vi "xy_graph_copy_format-vertical.vi"(6 "xy_scales_to_copy":i32=1, 8 "error in (no error)":errorcluster, 10 "destination":refnum<vi>, 11 "source":refnum<vi>) -> (0 "error out":errorcluster)   [LabVIEW 2015, in "lv-graph.lvlib"]
uses:
  lv-graph.lvlib
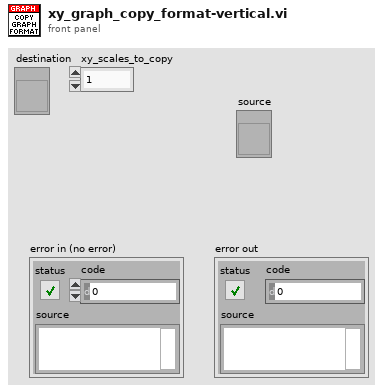
[diagram p1: front panel]
types:
  T1 = typedef "LVRangeTypeDef.ctl" = cluster{"Minimum":dbl, "Maximum":dbl, "Increment":dbl, "Minor Increment":dbl, "Start":dbl}
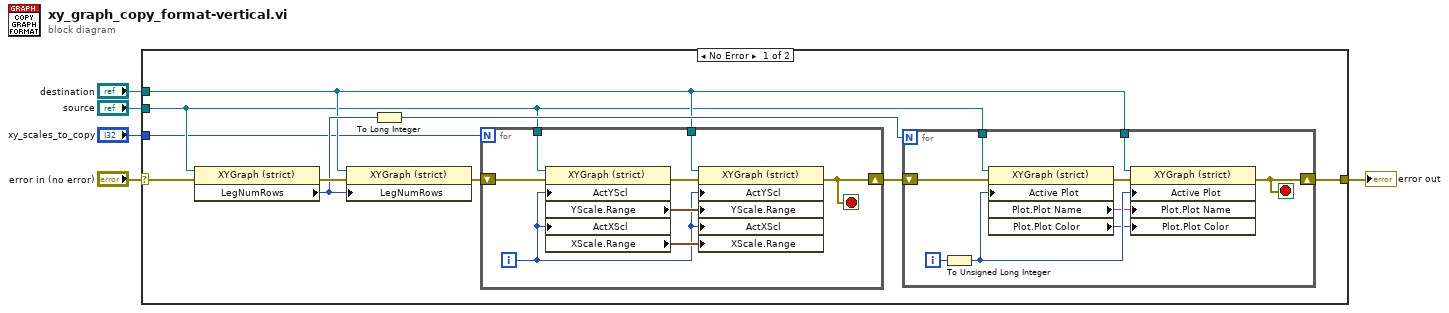
[diagram p0: block diagram]
diagram:
  n1 = case shown="No Error" "error in (no error)" {
    selector: "error in (no error)" -> [w7 w33]
    tunnel: [w12 w33] -> w5
    tunnel: "destination" -> [w9 _]
    tunnel: "source" -> [w8 _]
    tunnel: "xy_scales_to_copy" -> [w6 _]
    frame No Error {
      n2 = property class="XYGraph (strict)"(reference=w8, error in=w7) -> (error out=w15:errorcluster, "LegNumRows"=w14:u32)  [unwired: 1 out]
      n3 = property on="Property Node" class="XYGraph (strict)"(reference=w9, error in=w15, "LegNumRows"=w14) -> (error out=w11:errorcluster)  [unwired: 1 out]
      n4 = To Long Integer(number=w14) -> (32bit integer=w13:i32)
      n5 = for {
        N: w6 -> [_]
        shift-right: [w20] -> w10
        shift-left: w11 -> [w21]
        tunnel: w8 -> [w19]
        tunnel: w9 -> [w18]
        i -> [w16]
        stop <- w20 stop-if-true
        n6 = property on="Property Node" class="XYGraph (strict)"(reference=w19, error in=w21, "ActYScl"=w16, "ActXScl"=w16) -> (error out=w23:errorcluster, "YScale.Range"=w22:T1, "XScale.Range"=w17:T1)  [unwired: 1 out]
        n7 = property on="Property Node" class="XYGraph (strict)"(reference=w18, error in=w23, "ActYScl"=w16, "YScale.Range"=w22, "ActXScl"=w16, "XScale.Range"=w17) -> (error out=w20:errorcluster)  [unwired: 1 out]
      }
      n8 = for {
        N: w13 -> [_]
        shift-right: [w26] -> w12
        shift-left: w10 -> [w31]
        tunnel: w9 -> [w25]
        tunnel: w8 -> [w24]
        i -> [w30]
        stop <- w26 stop-if-true
        n9 = To Unsigned Long Integer(number=w30) -> (unsigned 32bit integer=w32:u32)
        n10 = property class="XYGraph (strict)"(reference=w24, error in=w31, "Active Plot"=w32) -> (error out=w29:errorcluster, "Plot.Plot Name"=w28:string, "Plot.Plot Color"=w27:u32)  [unwired: 1 out]
        n11 = property on="Property Node" class="XYGraph (strict)"(reference=w25, error in=w29, "Active Plot"=w32, "Plot.Plot Name"=w28, "Plot.Plot Color"=w27) -> (error out=w26:errorcluster)  [unwired: 1 out]
      }
    }
    frame Error {
    }
  }
  "error out" <- w5
